vi "Default Settings.vi"(8 "error in (no error)":errorcluster, 10 "Module.lvclass":refnum<class "Module.lvclass">, 11 "Fixture in":refnum<class "Fixture.lvclass">) -> (0 "error out":errorcluster, 2 "Module.lvclass 2":refnum<class "Module.lvclass">, 3 "Fixture out":refnum<class "Fixture.lvclass">)   [LabVIEW 2020, in "Fixture.lvclass"]
uses:
  Fixture.lvclass
  Module/Module.lvclass
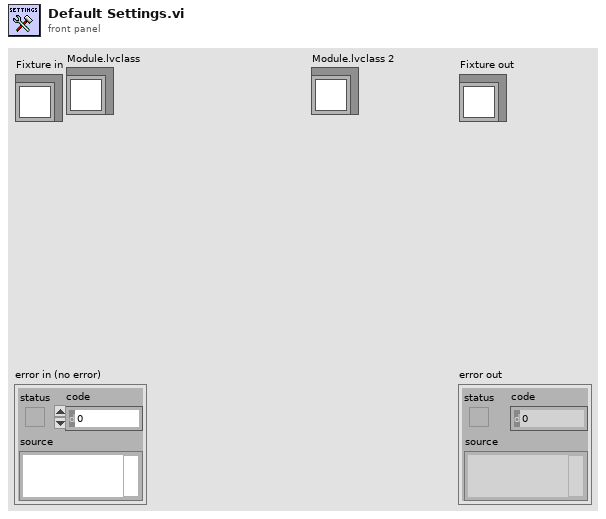
[diagram p1: front panel]
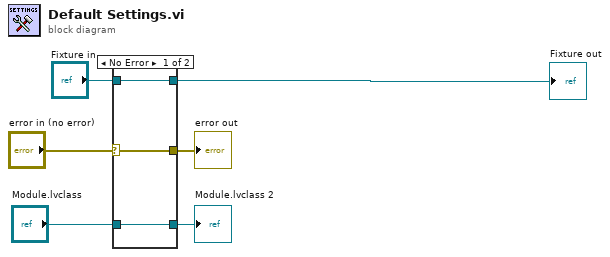
[diagram p0: block diagram]
diagram:
  n1 = case shown="No Error" "error in (no error)" {
    selector: "error in (no error)" -> [w9 w12]
    tunnel: [w9 w12] -> w5
    tunnel: [w7 w11] -> w3
    tunnel: "Fixture in" -> [w7 w11]
    tunnel: "Module.lvclass" -> [w8 w10]
    tunnel: [w8 w10] -> w2
    frame No Error {
    }
    frame Error {
    }
  }
  "error out" <- w5
  "Fixture out" <- w3
  "Module.lvclass 2" <- w2
